vi "ws_testing parse query string.vi"(11 "httpRequestID":u32) -> (0 "Client Address":string, 2 "TestSeqId":string, 3 "Action":string)   [LabVIEW 2011]
uses:
  <vilib>/addons/internet/utils/strutil.llb/Case Matching.ctl
  <vilib>/wsapi/NI_WebServices.lvlib
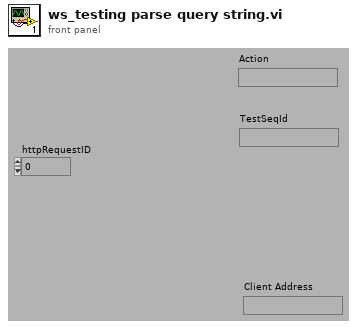
[diagram p1: front panel]
types:
  T1 = typedef "Case Matching.ctl" = enum16{"a != A", "a == A", "system"}
  T2 = typedef "Keyed Array.ctl" = cluster{"keys":string[], "values":string[]}
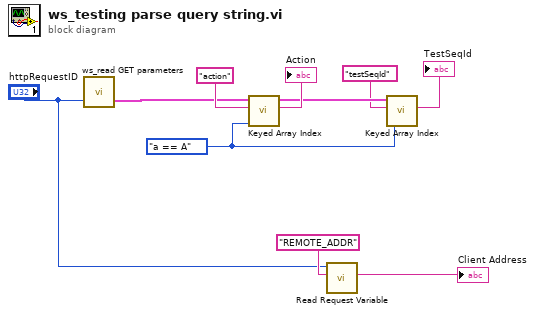
[diagram p0: block diagram]
diagram:
  w4 = Case_Matching."a == A" ("case matching (sensitive)")
  n1 = call "ws_read GET parameters.vi"("httpRequestID"="httpRequestID") -> ("GET query params"=w2:T2)  [unwired: 2 in]
  n2 = call <vilib>:"Keyed Array Index.vi"("case matching (sensitive)"=w4, "key"="action", "array in"=w2) -> ("value"=→"Action":string, "duplicate array"=w8:T2)  [unwired: 1 in, 2 out]
  n3 = call <vilib>:"Read Request Variable.vi"("variable name"="REMOTE_ADDR" ("key"), "httpRequestID"="httpRequestID") -> ("value"=→"Client Address":string)  [unwired: 7 in, 2 out]
  n4 = call <vilib>:"Keyed Array Index.vi"("case matching (sensitive)"=w4, "key"="testSeqId", "array in"=w8) -> ("value"=→"TestSeqId":string)  [unwired: 1 in, 3 out]
